vi "picoExtension.vi"() -> ()   [LabVIEW 2019]
uses:
  usbtc08.dll
panel:
  out "XY Graph 2":cluster{"X":dbl, "Y":dbl}[](graph)
  in  "?":bool
  in  "Ch # 8":bool
  in  "Type # 8":i16(ring)=107 items=["B"=98, "E"=101, "J"=106, "K"=107, "N"=110, "R"=114, "S"=115, "T"=116, "Voltage"=120]
  in  "Ch # 7":bool
  in  "Type # 7":i16(ring)=107 items=["B"=98, "E"=101, "J"=106, "K"=107, "N"=110, "R"=114, "S"=115, "T"=116, "Voltage"=120]
  in  "Ch # 6":bool
  in  "Type # 6":i16(ring)=107 items=["B"=98, "E"=101, "J"=106, "K"=107, "N"=110, "R"=114, "S"=115, "T"=116, "Voltage"=120]
  in  "Ch # 5":bool
  in  "Type # 5":i16(ring)=107 items=["B"=98, "E"=101, "J"=106, "K"=107, "N"=110, "R"=114, "S"=115, "T"=116, "Voltage"=120]
  in  "Ch # 4":bool
  in  "Type # 4":i16(ring)=107 items=["B"=98, "E"=101, "J"=106, "K"=107, "N"=110, "R"=114, "S"=115, "T"=116, "Voltage"=120]
  in  "Ch # 3":bool
  in  "Type # 3":i16(ring)=107 items=["B"=98, "E"=101, "J"=106, "K"=107, "N"=110, "R"=114, "S"=115, "T"=116, "Voltage"=120]
  in  "Ch# 2":bool=TRUE
  in  "Type # 2":i16(ring)=107 items=["B"=98, "E"=101, "J"=106, "K"=107, "N"=110, "R"=114, "S"=115, "T"=116, "Voltage"=120]
  in  "Ch# 1":bool=TRUE
  in  "Type # 1":i16(ring)=107 items=["B"=98, "E"=101, "J"=106, "K"=107, "N"=110, "R"=114, "S"=115, "T"=116, "Voltage"=120]
  in  "Units":enum16{"C°", "F°", "K°", "R°"}(ring)
  in  "stop":bool
  out "?":dynamicdata(graph)
  out "Min Interval (ms)":i32
  out "3":sgl
  out "4":sgl
  out "Handle":i16
  in  "Mains Frequency":i16(ring) items=["50 Hz", "60 Hz"]
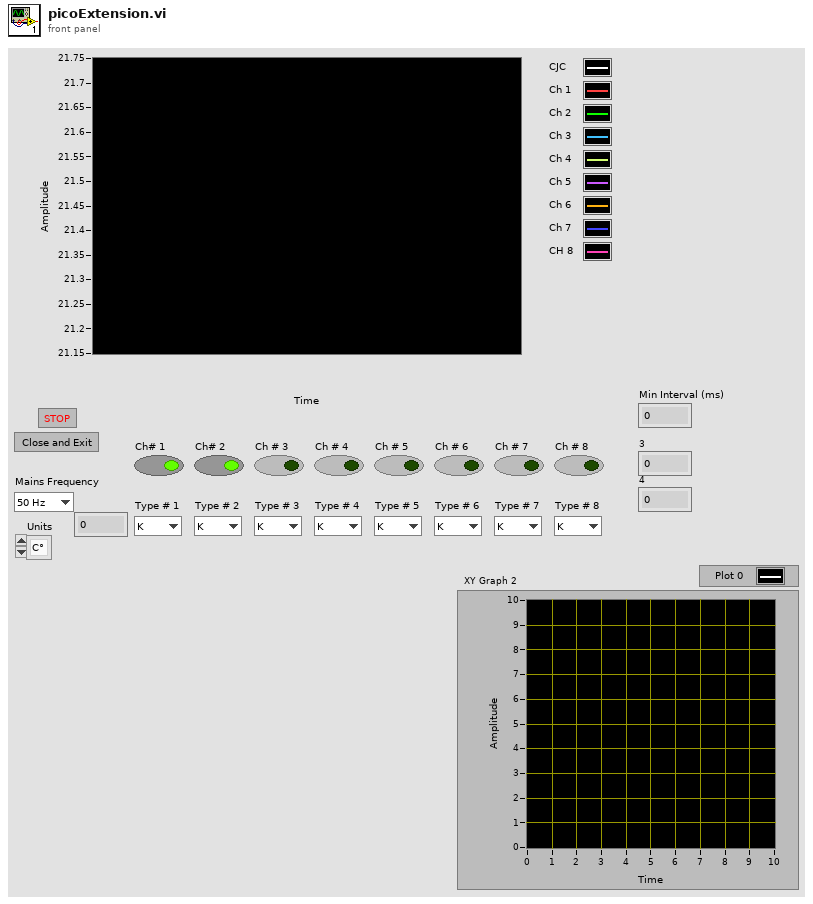
[diagram p1: front panel]
types:
  T1 = enum16{"open", "replace", "create", "open or create", "replace or create", "replace or create with confirmation"}
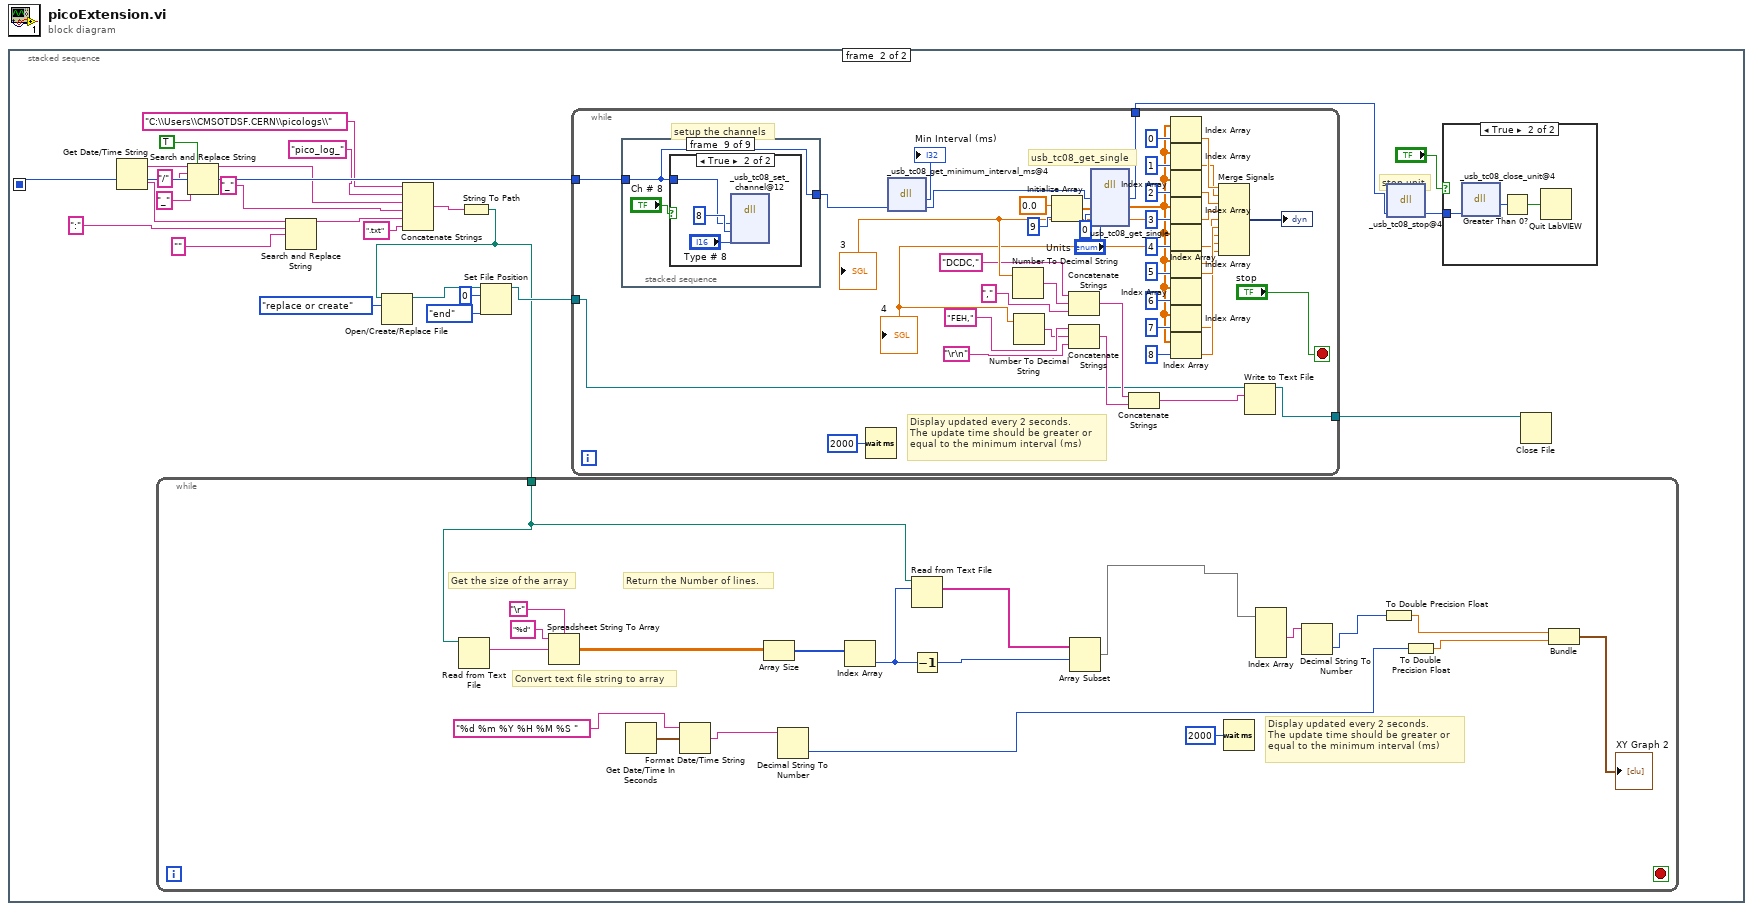
[diagram p0: block diagram]
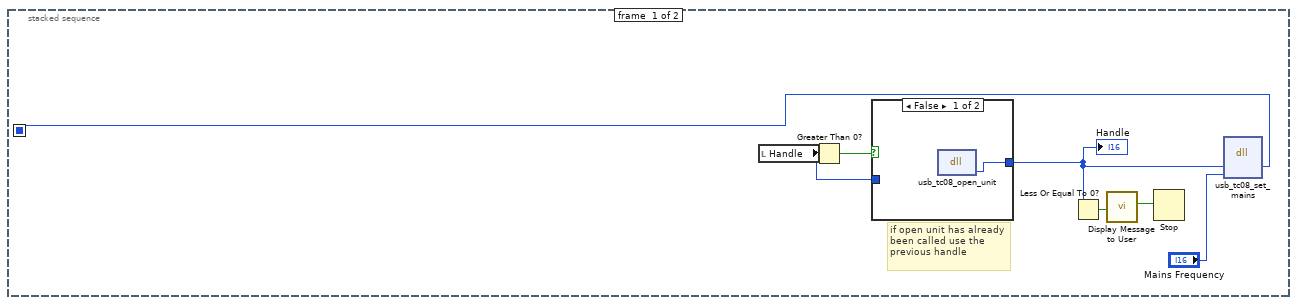
[diagram p2: hidden frame]
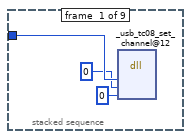
[diagram p4: hidden frame]
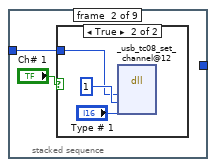
[diagram p5: hidden frame]
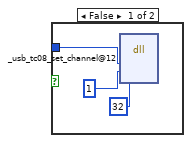
[diagram p6: hidden frame]
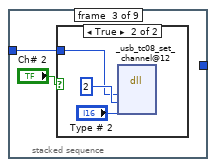
[diagram p7: hidden frame]
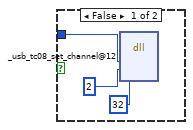
[diagram p8: hidden frame]
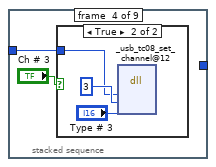
[diagram p9: hidden frame]
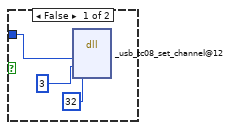
[diagram p10: hidden frame]
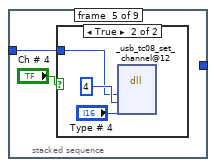
[diagram p11: hidden frame]
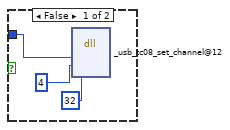
[diagram p12: hidden frame]
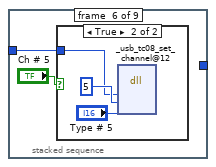
[diagram p13: hidden frame]
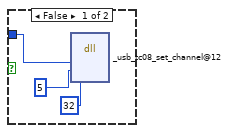
[diagram p14: hidden frame]
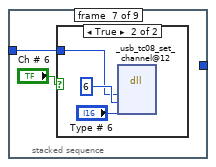
[diagram p15: hidden frame]
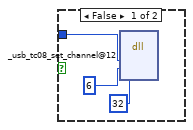
[diagram p16: hidden frame]
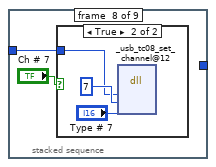
[diagram p17: hidden frame]
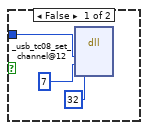
[diagram p18: hidden frame]
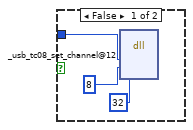
[diagram p19: hidden frame]
diagram:
  n1 = stacked-sequence {
    seq-local: [w5 _] -> [_ w34]
    frame #0 {
      # "if open unit has already been called use the previous handle"
      n2 = local read "Handle"() -> (w6:i16)
      n3 = Greater Than 0?(x=w6) -> (x > 0?=w7:bool)
      n4 = case shown="False" w7 {
        tunnel: [w8 w9] -> w4
        tunnel: w6 -> [_ w9]
        frame False {
          n5 = dll-call lib="usbtc08.dll" fn="usb_tc08_open_unit" label="OpenUnit"() -> ("Handle"=w8:i16)  [unwired: 3 in, 2 out]
        }
        frame True {
        }
      }
      "Handle" <- w4
      n6 = Less Or Equal To 0?(x=w4) -> (x <= 0?=w3:bool)
      n7 = call "Display Message to User"("Enable"=w3) -> ("OK"=w2:bool)  [unwired: 9 in, 1 out]
      n8 = Stop(stop? (T)=w2) -> ()
      n9 = dll-call lib="usbtc08.dll" fn="usb_tc08_set_mains" label="Set Mains"("Handle"=w4, "sixtyHertz"="Mains Frequency") -> ("Handle"=w5:i16)  [unwired: 5 in, 2 out]
    }
    frame #1 {
      # "stop unit"
      n10 = Get Date/Time String() -> (date string=w24:string, time string=w22:string)  [unwired: 3 in]
      n11 = Search and Replace String(replace all?=TRUE ("replace all? (F)"), input string=w24, search string="/", replace string="_" ("replace string (\"\")")) -> (result string=w23:string)  [unwired: 4 in, 3 out]
      n12 = Search and Replace String(input string=w22, search string=":", replace string="" ("replace string (\"\")")) -> (result string=w21:string)  [unwired: 5 in, 3 out]
      n13 = Concatenate Strings("C:\\Users\\CMSOTDSF.CERN\\picologs\\" ("string"), "pico_log_" ("string"), w23, "_" ("string"), w21, ".txt" ("string")) -> (w20:string)
      n14 = String To Path(string=w20) -> (path=w10:path)
      n15 = while {
        tunnel: w10 -> [w45]
        stop <- _ stop-if-true
        # "Convert text file string to array"
        # "Return the Number of lines."
        # "Get the size of the array"
        # "Display updated every 2 seconds.\nThe update time should be greater or\nequal to the minimum interval (ms)"
        n16 = Read from Text File(file (use dialog)=w45) -> (text=w50:string)  [unwired: 1 in, 5 out]
        n17 = Spreadsheet String To Array(delimiter (Tab)="\r", format string="%d", spreadsheet string=w50) -> (array=w48:dbl[][])  [unwired: 1 out]
        n18 = Get Date/Time In Seconds() -> (seconds since 1Jan1904=w43:timestamp)
        n19 = Format Date/Time String(time format string (%c)="%d %m %Y %H %M %S ", seconds (now)=w43) -> (date/time string=w40:string)  [unwired: 1 in]
        n20 = Array Size(array=w48) -> (size(s)=w49:i32[])
        n21 = Decimal String To Number(string=w40) -> (number=w38:i32)  [unwired: 2 in, 1 out]
        n22 = Index Array(array=w49) -> (element=w52:i32)  [unwired: 1 in]
        n23 = Read from Text File(file (use dialog)=w45, count=w52) -> (text=w53:string[])  [unwired: 1 in, 4 out]
        n24 = Decrement(x=w52) -> (x-1=w51:i32)
        n25 = Array Subset(array=w53, index=w51) -> (w44:string[])  [unwired: 1 in]
        n26 = Wait (ms)(milliseconds to wait=u32 2000) -> ()  [unwired: 1 out]
        n27 = Index Array(array=w44) -> (element #2=w41:string)  [unwired: 4 in, 3 out]
        n28 = Decimal String To Number(string=w41) -> (number=w39:i32)  [unwired: 2 in, 1 out]
        n29 = To Double Precision Float(number=w39) -> (double precision float=w37:dbl)
        n30 = To Double Precision Float(number=w38) -> (double precision float=w36:dbl)
        n31 = Bundle(w37, w36) -> (→"XY Graph 2":cluster{dbl, dbl})  [unwired: 1 in]
      }
      n32 = Open/Create/Replace File(file path (use dialog)=w10, operation (0:open)=T1."replace or create") -> (refnum out=w30:refnum<file>)  [unwired: 4 in, 2 out]
      n33 = Set File Position(offset (in bytes) (0)=i64 0, refnum=w30, from (0:start)=enum16{"start", "end", "current"}."end") -> (refnum out=w26:refnum<file>)  [unwired: 1 in, 1 out]
      n34 = while {
        tunnel: w34 -> [w97]
        tunnel: [w74] -> w31
        tunnel: w26 -> [w56]
        tunnel: [w55] -> w25
        stop <- "stop" stop-if-true
        # "Display updated every 2 seconds.\nThe update time should be greater or\nequal to the minimum interval (ms)"
        # "usb_tc08_get_single"
        # "setup the channels"
        n35 = stacked-sequence {
          tunnel: w97 -> [w100 w102 w110 w118 w126 w134 w142 w150 w157]
          tunnel: [_ _ _ _ _ _ _ _ w157] -> w70
          frame #0 {
            n36 = dll-call lib="usbtc08.dll" fn="_usb_tc08_set_channel@12"("handle"=w100, "channel"=i16 0, "tc_type"=i8 0) -> ()  [unwired: 7 in, 2 out]
          }
          frame #1 {
            n37 = case shown="True" "Ch# 1" {
              tunnel: w102 -> [w104 w107]
              frame False {
                n38 = dll-call lib="usbtc08.dll" fn="_usb_tc08_set_channel@12"("handle"=w104, "channel"=i16 1, "tc_type"=32) -> ()  [unwired: 7 in, 2 out]
              }
              frame True {
                n39 = dll-call lib="usbtc08.dll" fn="_usb_tc08_set_channel@12"("handle"=w107, "channel"=i16 1, "tc_type"="Type # 1") -> ()  [unwired: 7 in, 2 out]
              }
            }
          }
          frame #2 {
            n40 = case shown="True" "Ch# 2" {
              tunnel: w110 -> [w111 w115]
              frame False {
                n41 = dll-call lib="usbtc08.dll" fn="_usb_tc08_set_channel@12"("handle"=w111, "channel"=i16 2, "tc_type"=32) -> ()  [unwired: 7 in, 2 out]
              }
              frame True {
                n42 = dll-call lib="usbtc08.dll" fn="_usb_tc08_set_channel@12"("handle"=w115, "channel"=i16 2, "tc_type"="Type # 2") -> ()  [unwired: 7 in, 2 out]
              }
            }
          }
          frame #3 {
            n43 = case shown="True" "Ch # 3" {
              tunnel: w118 -> [w119 w123]
              frame False {
                n44 = dll-call lib="usbtc08.dll" fn="_usb_tc08_set_channel@12"("handle"=w119, "channel"=i16 3, "tc_type"=32) -> ()  [unwired: 7 in, 2 out]
              }
              frame True {
                n45 = dll-call lib="usbtc08.dll" fn="_usb_tc08_set_channel@12"("handle"=w123, "channel"=i16 3, "tc_type"="Type # 3") -> ()  [unwired: 7 in, 2 out]
              }
            }
          }
          frame #4 {
            n46 = case shown="True" "Ch # 4" {
              tunnel: w126 -> [w127 w131]
              frame False {
                n47 = dll-call lib="usbtc08.dll" fn="_usb_tc08_set_channel@12"("handle"=w127, "channel"=i16 4, "tc_type"=32) -> ()  [unwired: 7 in, 2 out]
              }
              frame True {
                n48 = dll-call lib="usbtc08.dll" fn="_usb_tc08_set_channel@12"("handle"=w131, "channel"=i16 4, "tc_type"="Type # 4") -> ()  [unwired: 7 in, 2 out]
              }
            }
          }
          frame #5 {
            n49 = case shown="True" "Ch # 5" {
              tunnel: w134 -> [w135 w139]
              frame False {
                n50 = dll-call lib="usbtc08.dll" fn="_usb_tc08_set_channel@12"("handle"=w135, "channel"=i16 5, "tc_type"=32) -> ()  [unwired: 7 in, 2 out]
              }
              frame True {
                n51 = dll-call lib="usbtc08.dll" fn="_usb_tc08_set_channel@12"("handle"=w139, "channel"=i16 5, "tc_type"="Type # 5") -> ()  [unwired: 7 in, 2 out]
              }
            }
          }
          frame #6 {
            n52 = case shown="True" "Ch # 6" {
              tunnel: w142 -> [w143 w147]
              frame False {
                n53 = dll-call lib="usbtc08.dll" fn="_usb_tc08_set_channel@12"("handle"=w143, "channel"=i16 6, "tc_type"=32) -> ()  [unwired: 7 in, 2 out]
              }
              frame True {
                n54 = dll-call lib="usbtc08.dll" fn="_usb_tc08_set_channel@12"("handle"=w147, "channel"=i16 6, "tc_type"="Type # 6") -> ()  [unwired: 7 in, 2 out]
              }
            }
          }
          frame #7 {
            n55 = case shown="True" "Ch # 7" {
              tunnel: w150 -> [w151 w155]
              frame False {
                n56 = dll-call lib="usbtc08.dll" fn="_usb_tc08_set_channel@12"("handle"=w151, "channel"=i16 7, "tc_type"=32) -> ()  [unwired: 7 in, 2 out]
              }
              frame True {
                n57 = dll-call lib="usbtc08.dll" fn="_usb_tc08_set_channel@12"("handle"=w155, "channel"=i16 7, "tc_type"="Type # 7") -> ()  [unwired: 7 in, 2 out]
              }
            }
          }
          frame #8 {
            n58 = case shown="True" "Ch # 8" {
              tunnel: w157 -> [w159 w163]
              frame False {
                n59 = dll-call lib="usbtc08.dll" fn="_usb_tc08_set_channel@12"("handle"=w159, "channel"=i16 8, "tc_type"=32) -> ()  [unwired: 7 in, 2 out]
              }
              frame True {
                n60 = dll-call lib="usbtc08.dll" fn="_usb_tc08_set_channel@12"("handle"=w163, "channel"=i16 8, "tc_type"="Type # 8") -> ()  [unwired: 7 in, 2 out]
              }
            }
          }
        }
        n61 = Wait (ms)(milliseconds to wait=u32 2000) -> ()  [unwired: 1 out]
        n62 = dll-call lib="usbtc08.dll" fn="_usb_tc08_get_minimum_interval_ms@4"("handle"=w70) -> ("Min Interval (ms)"=→"Min Interval (ms)":i32, "handle"=w69:i16)  [unwired: 3 in, 2 out]
        n63 = Initialize Array(sgl 0.0, i16 9) -> (w96:sgl[])
        n64 = dll-call lib="usbtc08.dll" fn="usb_tc08_get_single"("handle"=w69, "temp_buffer"=w96, "overflow"=i16 0, "units"="Units") -> ("handle"=w74:i16, "temp_buffer"=w82:sgl[])  [unwired: 6 in, 2 out]
        n65 = Index Array(array=w82, index=i16 0) -> (element=w81:sgl)
        n66 = Index Array(array=w82, index=i16 1) -> (element=w73:sgl)
        n67 = Index Array(array=w82, index=i16 2) -> (element=w80:sgl)
        n68 = Index Array(array=w82, index=i16 3) -> (element=w67:sgl)
        "3" <- w67
        n69 = Number To Decimal String(number=w67) -> (decimal integer string=w63:string)  [unwired: 1 in]
        n70 = Concatenate Strings("DCDC,", w63, ",") -> (w59:string)
        n71 = Index Array(array=w82, index=4) -> (element=w66:sgl)
        "4" <- w66
        n72 = Number To Decimal String(number=w66) -> (decimal integer string=w61:string)  [unwired: 1 in]
        n73 = Concatenate Strings("FEH,", w61, "\r\n") -> (w58:string)
        n74 = Concatenate Strings(w59, w58) -> (w57:string)
        n75 = Index Array(array=w82, index=i16 5) -> (element=w79:sgl)
        n76 = Index Array(array=w82, index=6) -> (element=w78:sgl)
        n77 = Index Array(array=w82, index=i16 7) -> (element=w76:sgl)
        n78 = Index Array(array=w82, index=i16 8) -> (element=w77:sgl)
        n79 = Merge Signals(w81, w73, w80, w67, w66, w79, w78, w76, w77) -> (→"?":dynamicdata)
        n80 = Write to Text File(file (use dialog)=w56, text=w57) -> (refnum out=w55:refnum<file>)  [unwired: 2 in, 2 out]
      }
      n81 = dll-call lib="usbtc08.dll" fn="_usb_tc08_stop@4" ("Close unit")("handle"=w31) -> ("handle"=w33:i16)  [unwired: 4 in, 2 out]
      n82 = case shown="True" "?" {
        tunnel: w33 -> [_ w167]
        frame False {
        }
        frame True {
          n83 = dll-call lib="usbtc08.dll" fn="_usb_tc08_close_unit@4" ("Close unit")("handle"=w167) -> ("return type"=w166:i16)  [unwired: 4 in, 2 out]
          n84 = Greater Than 0?(x=w166) -> (x > 0?=w165:bool)
          n85 = Quit LabVIEW(quit? (T)=w165) -> ()
        }
      }
      n86 = Close File(refnum=w25) -> ()  [unwired: 1 in, 2 out]
    }
  }
